vi "DP-Transpose.vi"(5 "USER ID":string="ML", 7 "ANIMAL ID":i32=15, 9 "EAR":string="R", 11 "RUN":i32, 13 "Array of f2's":i32[](array[numeric])=[5660, 6730, 8000, 9520, 11300, 13460, 16000, 19040, 22650, 26920, 32000, 38050, 45200]) -> ()   [LabVIEW 2020]
uses:
  <vilib>/Analysis/NI_AALBase.lvlib
panel:
  out "ERROR":bool
  in  "Criterion for Database":u16(ring)=1 items=["-5 dB", "0 dB ", "5 dB", "10 dB"]
  in  "Return":bool
  in  "Start":bool
  out "File Error":bool
  in  "PARTITION":string="C:\\Data\\"
  out "FINAL GRAPH":cluster{dbl[], dbl[]}[](graph)=[{[5.6, 22.6, 32.0], [72.77611940298507, 24.79591836734694, 35.338770388958594]}, {[5.6, 8.0, 16.0, 22.6, 32.0, 45.2], [85.0, 75.33814247069432, 32.34341252699784, 29.006462035541194, 38.47553324968632, 45.006435006435005]}, {[5.6, 8.0, 11.3, 16.0, 22.6, 32.0, 45.2], [85.0, 77.59242560865644, 77.35252808988764, 37.61316872427984, 33.12603648424544, 42.6440329218107, 48.22393822393823]}, {[5.6, 8.0, 11.3, 16.0, 22.6, 32.0, 45.2], [85.0, 79.84670874661857, 85.0, 43.13084112149533, 37.5607476635514, 50.080906148867314, 51.63265306122449]}, {[5.6, 8.0, 11.3, 16.0, 22.6, 32.0, 45.2], [85.0, 85.0, 85.0, 49.28211586901763, 43.80573248407644, 70.90986394557824, 55.329861111111114]}, {[5.6, 8.0, 11.3, 16.0, 22.6, 32.0, 45.2], [85.0, 85.0, 85.0, 57.552742616033754, 66.34316770186335, 72.32709750566893, 59.67013888888889]}, {[5.6, 8.0, 11.3, 16.0, 22.6, 32.0, 45.2], [85.0, 85.0, 85.0, 64.66019417475728, 70.18613607188703, 73.74433106575964, 65.31879194630872]}]
  in  "Which DP":bool=TRUE
  out "I-O GRAPH":cluster{ext[], ext[]}[](graph)=[{[10.0, 15.0, 20.0, 25.0, 30.0, 35.0, 40.0, 45.0, 50.0, 55.0, 60.0, 65.0, 70.0, 75.0, 80.0], [-21.38, -4.92, -4.57, -12.49, -18.58, -19.55, -10.63, -13.68, -10.35, -11.85, -9.81, -9.89, -6.86, -3.51, -9.21]}, {[10.0, 15.0, 20.0, 25.0, 30.0, 35.0, 40.0, 45.0, 50.0, 55.0, 60.0, 65.0, 70.0, 75.0, 80.0], [-12.46, -6.43, -7.62, 0.71, -8.47, -7.75, -3.16, -1.91, -3.14, -2.22, -12.37, -7.72, -2.6, -0.75, 10.34]}, {[10.0, 15.0, 20.0, 25.0, 30.0, 35.0, 40.0, 45.0, 50.0, 55.0, 60.0, 65.0, 70.0, 75.0, 80.0], [-9.79, -1.17, -1.26, 8.27, -8.03, -2.71, -6.35, -10.3, -1.88, -1.74, 0.93, 4.21, 2.16, 1.65, 8.77]}, {[10.0, 15.0, 20.0, 25.0, 30.0, 35.0, 40.0, 45.0, 50.0, 55.0, 60.0, 65.0, 70.0, 75.0, 80.0], [-6.83, -9.43, -10.07, -8.11, -2.17, 2.46, 7.32, 11.6, 15.57, 18.79, 21.16, 25.28, 30.33, 35.66, 37.1]}, {[10.0, 15.0, 20.0, 25.0, 30.0, 35.0, 40.0, 45.0, 50.0, 55.0, 60.0, 65.0, 70.0, 75.0, 80.0], [-9.81, -5.62, -5.94, -4.96, 1.23, 7.26, 12.61, 15.75, 17.7, 18.3, 18.08, 18.27, 24.71, 32.5, 37.52]}, {[10.0, 15.0, 20.0, 25.0, 30.0, 35.0, 40.0, 45.0, 50.0, 55.0, 60.0, 65.0, 70.0, 75.0, 80.0], [-7.23, -10.81, -18.72, -21.87, -8.97, -5.54, 2.43, 7.29, 9.95, 13.04, 14.52, 12.51, 11.79, 29.43, 37.82]}, {[10.0, 15.0, 20.0, 25.0, 30.0, 35.0, 40.0, 45.0, 50.0, 55.0, 60.0, 65.0, 70.0, 75.0, 80.0], [-1.57, -13.83, -4.88, -2.53, -4.33, -8.02, -2.22, -0.01, 7.76, 14.62, 20.38, 24.81, 27.79, 30.32, 31.98]}]
  in  "?":ext[](array[numeric]) format="%.2f"
  out "?":string="5645\t-10.9\t2.6\r7995\t-5.6\t2.3\r11322\t-4.1\t4.1\r15991\t-8.0\t3.2\r22644\t-8.5\t1.6\r32012\t-10.4\t2.7\r45257\t-5.0\t2.4\r"
  # "85 dB means DP never reaches criterion"
  # "Nse Flr"
  # "f2 (Hz)"
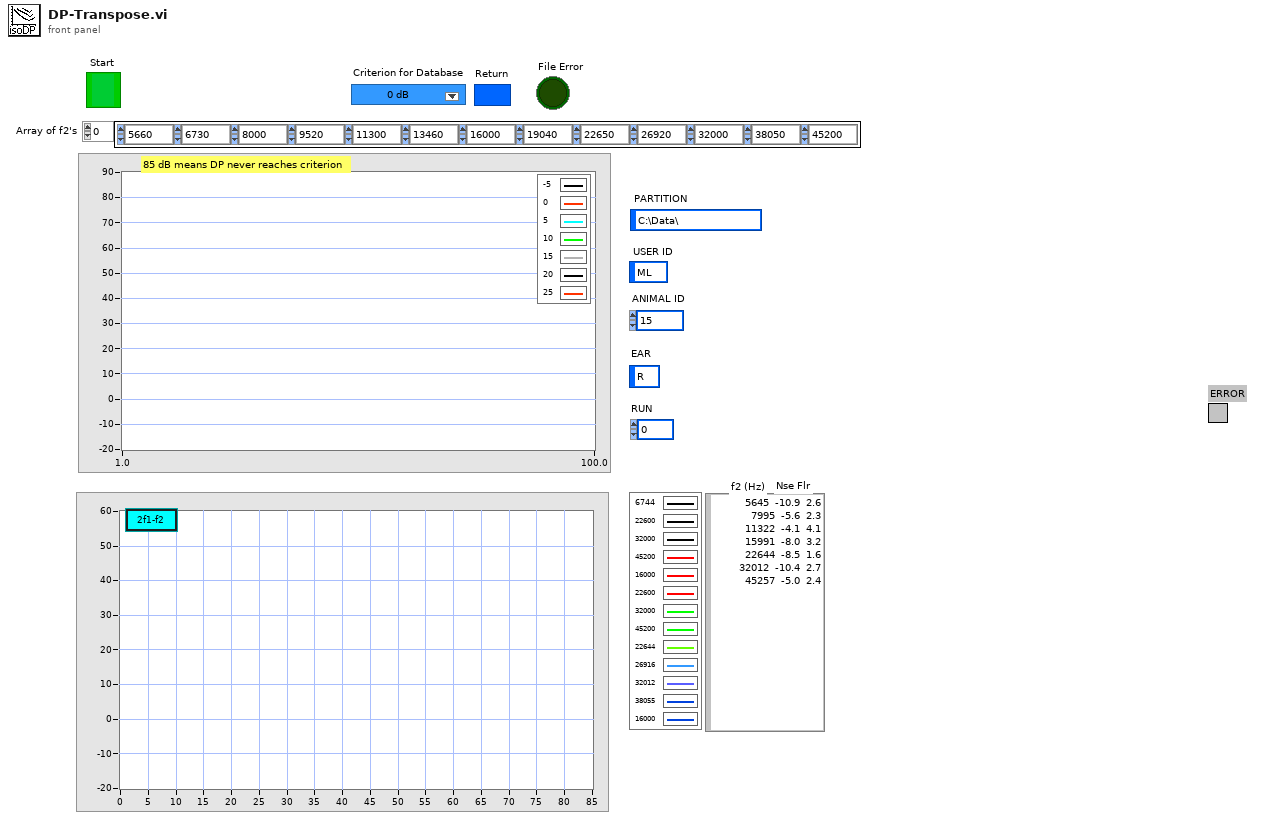
[diagram p1: front panel]
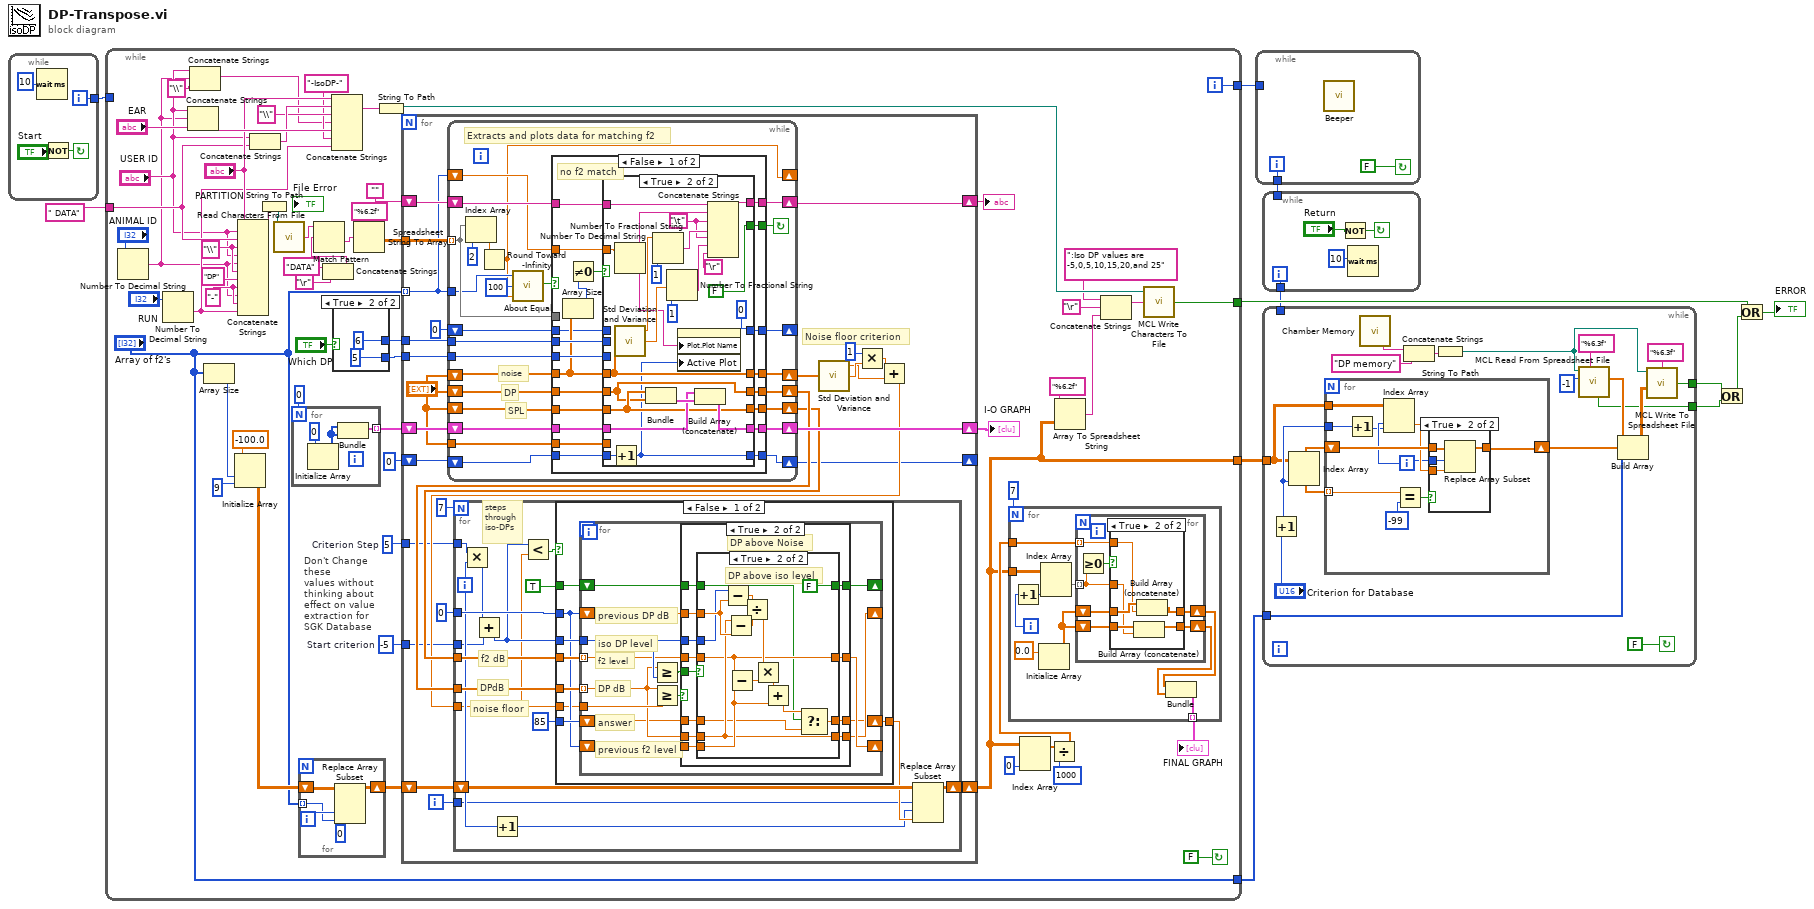
[diagram p0: block diagram]
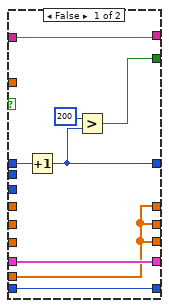
[diagram p4: hidden frame]
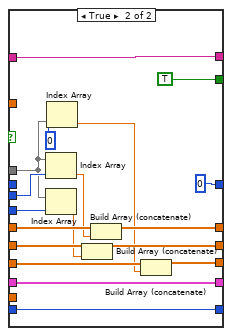
[diagram p5: hidden frame]
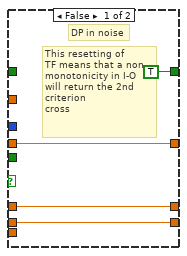
[diagram p6: hidden frame]
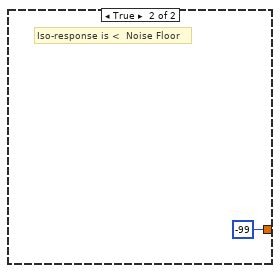
[diagram p8: hidden frame]
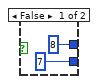
[diagram p9: hidden frame]
diagram:
  n1 = while {
    tunnel: [w16] -> w12
    i -> [w16]
    stop <- w14 continue-if-true
    n2 = Wait (ms)(milliseconds to wait=10) -> ()  [unwired: 1 out]
    n3 = Not(x="Start") -> (.not. x?=w14:bool)
  }
  n4 = while {
    tunnel: " DATA" -> [w29]
    tunnel: [w30] -> w4
    tunnel: w12 -> [_]
    tunnel: [w22] -> w10
    tunnel: [w17] -> w9
    tunnel: ["Array of f2's"] -> w1
    i -> [w30]
    stop <- FALSE continue-if-true
    w38 = 5  # Criterion Step
    w39 = -5  # Start criterion
    w71 = "-"
    w73 = "\\"
    # "Don't Change these\nvalues without thinking about\neffect on value extraction for\nSGK Database"
    n5 = Number To Decimal String(number="ANIMAL ID") -> (decimal integer string=w26:string)  [unwired: 1 in]
    n6 = Number To Decimal String(number="RUN") -> (decimal integer string=w28:string)  [unwired: 1 in]
    n7 = Concatenate Strings("USER ID", w26, "EAR") -> (w44:string)
    n8 = Concatenate Strings("USER ID", w26, "\\") -> (w24:string)
    n9 = Array Size(array="Array of f2's") -> (size(s)=w61:i32)
    n10 = Initialize Array(-100.0, w61, 9) -> (w57:dbl[][])
    n11 = Concatenate Strings("PARTITION", "USER ID", w29, w73, "USER ID", w26, w73, "DP", w71, w26, w71, w28) -> (w34:string)
    n12 = Concatenate Strings("USER ID", w29) -> (w42:string)
    n13 = String To Path(string=w34) -> (path=w70:path)
    n14 = call <vilib>:"Read Characters From File.vi"("file path (dialog if empty)"=w70) -> ("character string"=w33:string)  [unwired: 5 in, 3 out]
    n15 = for {
      N: 0 -> [_]
      tunnel: [w309] -> w63 mode=indexing
      n16 = Initialize Array(0) -> (w310:i32[])  [unwired: 1 in]
      n17 = Bundle(w310, w310) -> (w309:cluster{i32[], i32[]})  [unwired: 1 in]
    }
    n18 = for {
      shift-right: [w105] -> w58
      shift-left: w57 -> [w106]
      tunnel: "Array of f2's" -> [w102] mode=indexing
      i -> [w103]
      n19 = Replace Array Subset(array=w106, new element=w102, index (row)=w103, index (col)=0) -> (w105:dbl[][])
    }
    n20 = Concatenate Strings("DATA", "\r") -> (w35:string)
    n21 = Match Pattern(string=w33, regular expression=w35) -> (after substring=w32:string)  [unwired: 1 in, 3 out]
    n22 = Concatenate Strings("PARTITION", w42, "\\", w24, w44, "-IsoDP-", w28) -> (w23:string)
    n23 = case shown="True" "Which DP" {
      tunnel: [7 5] -> w76
      tunnel: [8 6] -> w75
      frame False {
      }
      frame True {
      }
    }
    n24 = Spreadsheet String To Array(format string="%6.2f", spreadsheet string=w32) -> (array=w21:dbl[][])  [unwired: 2 in]
    n25 = String To Path(string=w23) -> (path=w49:path)
    n26 = for {
      tunnel: w21 -> [w133]
      tunnel: w75 -> [w132]
      tunnel: w76 -> [w131]
      tunnel: "Array of f2's" -> [w110] mode=indexing
      shift-right: [w129] -> w59
      shift-left: "" -> [w130]
      shift-right: [w128] -> w64
      shift-left: w63 -> [w127]
      shift-right: [w123] -> w22
      shift-left: w58 -> [w124]
      tunnel: w39 -> [w113]
      tunnel: w38 -> [w112]
      shift-right: [w108] -> _
      shift-left: 0 -> [w109]
      i -> [w121]
      # "Noise floor criterion"
      n27 = while {
        shift-left: 0 -> [w137]
        shift-right: [w138] -> _
        shift-left: w110 -> [w142]
        shift-right: [w136] -> _
        tunnel: w110 -> [w140]
        shift-left: w127 -> [w145]
        shift-right: [w144] -> w128
        shift-left: w130 -> [w147]
        shift-right: [w148] -> w129
        tunnel: "?" -> [w149]
        tunnel: w131 -> [w150]
        tunnel: w132 -> [w151]
        shift-left: "?" -> [w153]
        shift-right: [w154] -> w120
        shift-left: "?" -> [w155]
        shift-right: [w156] -> w122
        shift-left: "?" -> [w157]
        shift-right: [w158] -> w119
        tunnel: w133 -> [w152] mode=indexing
        shift-right: [w135] -> w108
        shift-left: w109 -> [w134]
        stop <- w143 continue-if-true
        # "Extracts and plots data for matching f2"
        # "SPL"
        # "DP"
        # "noise"
        n28 = Index Array(array=w152, index=2) -> (element=w146:dbl)
        n29 = Round Toward -Infinity(1:w146) -> (0:w136:dbl)
        n30 = call "About Equal.vi"("Standard Value"=w136, "+/- Range"=100, "Input Value"=w140) -> ("In Range?"=w141:bool)
        n31 = case shown="False" w141 {
          tunnel: [w171 w222] -> w158
          tunnel: w157 -> [w165 w221]
          tunnel: [w172 w223] -> w156
          tunnel: w155 -> [w177 w220]
          tunnel: [w174 w224] -> w154
          tunnel: w153 -> [w178 w219]
          tunnel: w152 -> [_ w226]
          tunnel: w151 -> [w168 w228]
          tunnel: w150 -> [w169 w227]
          tunnel: w149 -> [w173 _]
          tunnel: [w180 w215] -> w148
          tunnel: w147 -> [w179 w215]
          tunnel: w145 -> [w176 w214]
          tunnel: [w175 w214] -> w144
          tunnel: [w170 TRUE] -> w143
          tunnel: w142 -> [w164 _]
          tunnel: [w163 0] -> w138
          tunnel: w137 -> [w162 _]
          tunnel: [w161 w211] -> w135
          tunnel: w134 -> [w160 w211]
          frame False {
            # "no f2 match"
            n32 = Array Size(array=w165) -> (size(s)=w167:i32)
            n33 = Not Equal To 0?(x=w167) -> (x != 0?=w166:bool)
            n34 = case shown="True" w166 {
              tunnel: [w187 w207] -> w175
              tunnel: w176 -> [w187 w206]
              tunnel: w177 -> [_ w201]
              tunnel: w178 -> [_ w202]
              tunnel: w179 -> [w188 w204]
              tunnel: [w188 w205] -> w180
              tunnel: w165 -> [_ w200]
              tunnel: [w186 w202] -> w174
              tunnel: w173 -> [w186 _]
              tunnel: [w186 w201] -> w172
              tunnel: [w186 w200] -> w171
              tunnel: [w183 FALSE] -> w170
              tunnel: w169 -> [_ _]
              tunnel: w168 -> [_ _]
              tunnel: w164 -> [_ w192]
              tunnel: [w184 0] -> w163
              tunnel: w162 -> [w185 _]
              tunnel: [w181 w190] -> w161
              tunnel: w160 -> [w181 w191]
              frame False {
                n35 = Increment(x=w185) -> (x+1=w184:i32)
                n36 = Greater?(x=200, y=w184) -> (0:w183:bool)
              }
              frame True {
                w196 = "\t"
                n37 = Increment(x=w191) -> (x+1=w190:i32)
                n38 = Number To Decimal String(number=w192) -> (decimal integer string=w189:string)  [unwired: 1 in]
                n39 = call <vilib>:"Std Deviation and Variance.vi"("X"=w200) -> ("mean"=w199:dbl, "standard deviation"=w197:dbl)  [unwired: 1 in, 1 out]
                n40 = Bundle(w202, w201) -> (w210:cluster{ext[], ext[]})  [unwired: 1 in]
                n41 = Number To Fractional String(number=w199, precision (6)=1) -> (F-format string=w209:string)  [unwired: 2 in]
                n42 = Number To Fractional String(number=w197, precision (6)=1) -> (F-format string=w195:string)  [unwired: 2 in]
                n43 = property on="I-O GRAPH" class="XYGraph (strict)"("Plot.Plot Name"=w189, "Active Plot"=w190) -> ()  [unwired: 2 in, 2 out]
                n44 = Build Array (concatenate)(w206, w210) -> (w207:cluster{ext[], ext[]}[])
                n45 = Concatenate Strings(w204, w189, w196, w209, w196, w195, "\r") -> (w205:string)
              }
            }
          }
          frame True {
            # "f2 match"
            n46 = Index Array(array=w226, index=w228) -> (element=w217:dbl)
            n47 = Index Array(array=w226, index=w227) -> (element=w216:dbl)
            n48 = Index Array(array=w226, index=0) -> (element=w218:dbl)
            n49 = Build Array (concatenate)(w220, w216) -> (w223:ext[])
            n50 = Build Array (concatenate)(w221, w217) -> (w222:ext[])
            n51 = Build Array (concatenate)(w219, w218) -> (w224:ext[])
          }
        }
      }
      n52 = call <vilib>:"Std Deviation and Variance.vi"("X"=w119) -> ("mean"=w115:dbl, "standard deviation"=w118:dbl)  [unwired: 1 in, 1 out]
      n53 = Multiply(x=1, y=w118) -> (x*y=w116:dbl)
      n54 = Add(x=w116, y=w115) -> (x+y=w114:dbl)
      n55 = for {
        N: 7 -> [_]
        tunnel: w114 -> [w229]
        tunnel: 0 -> [w245]
        tunnel: w122 -> [w244]
        shift-right: [w238] -> w123
        shift-left: w124 -> [w240]
        tunnel: w121 -> [w236]
        tunnel: w120 -> [w243]
        tunnel: w113 -> [w233]
        tunnel: w112 -> [w232]
        i -> [w239]
        # "noise floor"
        # "DPdB"
        # "f2 dB"
        # "steps through iso-DPs"
        n56 = Multiply(x=w232, y=w239) -> (x*y=w242:i32)
        n57 = Add(x=w242, y=w233) -> (x+y=w230:i32)
        n58 = Increment(x=w239) -> (x+1=w235:i32)
        n59 = Less?(x=w230, y=w229) -> (x < y?=w231:bool)
        n60 = case shown="False" w231 {
          tunnel: TRUE -> [w253 _]
          tunnel: [w252 -99] -> w237
          tunnel: 85 -> [w251 _]
          tunnel: w230 -> [w250 _]
          tunnel: w243 -> [w249 _]
          tunnel: w244 -> [w248 _]
          tunnel: w245 -> [w247 _]
          tunnel: w229 -> [w246 _]
          frame False {
            n61 = for {
              tunnel: w248 -> [w258] mode=indexing
              tunnel: w246 -> [w267]
              shift-right: [w264] -> _
              shift-left: w247 -> [w261]
              shift-right: [w263] -> _
              shift-left: w247 -> [w262]
              tunnel: w250 -> [w260]
              tunnel: w249 -> [w259] mode=indexing
              shift-right: [w256] -> w252
              shift-left: w251 -> [w257]
              shift-right: [w255] -> _
              shift-left: w253 -> [w254]
              # "DP dB"
              # "f2 level"
              # "answer"
              # "iso DP level"
              # "previous f2 level"
              # "previous DP dB"
              n62 = Greater Or Equal?(x=w258, y=w260) -> (x >= y?=w266:bool)
              n63 = Greater Or Equal?(x=w258, y=w267) -> (x >= y?=w265:bool)
              n64 = case shown="True" w265 {
                tunnel: w266 -> [_ w276]
                tunnel: w259 -> [w270 w283]
                tunnel: w258 -> [w271 w282]
                tunnel: [w270 w280] -> w264
                tunnel: [w271 w281] -> w263
                tunnel: w260 -> [_ w279]
                tunnel: w262 -> [_ w278]
                tunnel: w261 -> [_ w277]
                tunnel: w257 -> [w269 w274]
                tunnel: [w269 w275] -> w256
                tunnel: [TRUE w273] -> w255
                tunnel: w254 -> [_ w272]
                frame False {
                  # "This resetting of\nTF means that a non-\nmonotonicity in I-O\nwill return the 2nd\ncriterion\ncross"
                  # "DP in noise"
                }
                frame True {
                  # "DP above Noise"
                  n65 = case shown="True" w276 {
                    tunnel: w283 -> [w287 w293]
                    tunnel: w282 -> [w286 w294]
                    tunnel: [w286 w294] -> w281
                    tunnel: [w287 w293] -> w280
                    tunnel: w279 -> [_ w295]
                    tunnel: w278 -> [_ w296]
                    tunnel: w277 -> [_ w302]
                    tunnel: [w285 w291] -> w275
                    tunnel: w274 -> [w285 w289]
                    tunnel: [w284 FALSE] -> w273
                    tunnel: w272 -> [w284 w288]
                    frame False {
                      # "DP too small"
                    }
                    frame True {
                      # "DP above iso level"
                      n66 = Subtract(x=w295, y=w296) -> (x-y=w297:ext)
                      n67 = Subtract(x=w294, y=w296) -> (x-y=w298:ext)
                      n68 = Subtract(x=w293, y=w302) -> (x-y=w300:ext)
                      n69 = Divide(x=w297, y=w298) -> (x/y=w299:ext)
                      n70 = Multiply(x=w299, y=w300) -> (x*y=w301:ext)
                      n71 = Add(x=w301, y=w302) -> (x+y=w290:ext)
                      n72 = Select(t=w290, s=w288, f=w289) -> (s? t:f=w291:ext)
                    }
                  }
                }
              }
            }
          }
          frame True {
            # "Iso-response is <  Noise Floor"
          }
        }
        n73 = Replace Array Subset(array=w240, new element=w237, index (row)=w236, index (col)=w235) -> (w238:dbl[][])
      }
    }
    "I-O GRAPH" <- w64
    "?" <- w59
    n74 = Index Array(array=w22, index (col)=0) -> (element=w53:dbl[])  [unwired: 1 in]
    n75 = Divide(x=w53, y=1000) -> (x/y=w51:dbl[])
    n76 = for {
      N: 7 -> [_]
      tunnel: [w81] -> w55 mode=indexing
      tunnel: w22 -> [w80]
      tunnel: w51 -> [w77]
      i -> [w86]
      n77 = Increment(x=w86) -> (x+1=w83:i32)
      n78 = Initialize Array(0.0) -> (w78:dbl[])  [unwired: 1 in]
      n79 = Index Array(array=w80, index (col)=w83) -> (element=w85:dbl[])  [unwired: 1 in]
      n80 = for {
        shift-right: [w92] -> w82
        shift-left: w78 -> [w91]
        shift-right: [w90] -> w84
        shift-left: w78 -> [w89]
        tunnel: w85 -> [w87] mode=indexing
        tunnel: w77 -> [w88] mode=indexing
        n81 = Greater Or Equal To 0?(x=w87) -> (x >= 0?=w93:bool)
        n82 = case shown="True" w93 {
          tunnel: [w95 w100] -> w92
          tunnel: w91 -> [w95 w101]
          tunnel: [w94 w99] -> w90
          tunnel: w89 -> [w94 w98]
          tunnel: w88 -> [_ w97]
          tunnel: w87 -> [_ w96]
          frame False {
          }
          frame True {
            n83 = Build Array (concatenate)(w98, w96) -> (w99:dbl[])
            n84 = Build Array (concatenate)(w101, w97) -> (w100:dbl[])
          }
        }
      }
      n85 = Bundle(w82, w84) -> (w81:cluster{dbl[], dbl[]})  [unwired: 1 in]
    }
    "FINAL GRAPH" <- w55
    n86 = Array To Spreadsheet String(array=w22, 3:"%6.2f") -> (spreadsheet string=w47:string)  [unwired: 1 in]
    n87 = Concatenate Strings(":Iso DP values are -5,0,5,10,15,20,and 25", "\r", w47) -> (w48:string)
    n88 = call "MCL Write Characters To File.vi"("character string"=w48, "file path (dialog if empty)"=w49) -> ("Filewrite Error"=w17:bool)  [unwired: 2 in, 1 out]
  }
  n89 = while {
    tunnel: w4 -> [_]
    tunnel: [w312] -> w3
    i -> [w312]
    stop <- FALSE continue-if-true
    n90 = call "Beeper.vi"() -> ()  [unwired: 1 in]
  }
  n91 = while {
    tunnel: w3 -> [_]
    tunnel: [w313] -> w2
    i -> [w313]
    stop <- w315 continue-if-true
    n92 = Not(x="Return") -> (.not. x?=w315:bool)
    n93 = Wait (ms)(milliseconds to wait=10) -> ()  [unwired: 1 out]
  }
  n94 = while {
    tunnel: w10 -> [w318]
    tunnel: [w324] -> w6
    tunnel: [w317] -> w5
    tunnel: w2 -> [_]
    tunnel: w1 -> [w322]
    stop <- FALSE continue-if-true
    n95 = Increment(x="Criterion for Database") -> (x+1=w320:u16)
    n96 = Index Array(array=w318, index (col)=w320) -> (element=w319:dbl[])  [unwired: 1 in]
    n97 = for {
      shift-right: [w341] -> w321
      shift-left: w319 -> [w340]
      tunnel: w319 -> [w343] mode=indexing
      tunnel: w318 -> [w339]
      tunnel: w320 -> [w338]
      i -> [w336]
      n98 = Increment(x=w338) -> (x+1=w335:u16)
      n99 = Index Array(array=w339, index (row)=w336, index (col)=w335) -> (element=w337:dbl)
      n100 = Equal?(x=w343, y=-99) -> (x = y?=w342:bool)
      n101 = case shown="True" w342 {
        tunnel: [w345 w348] -> w341
        tunnel: w340 -> [w345 w349]
        tunnel: w336 -> [_ w347]
        tunnel: w337 -> [_ w346]
        frame False {
        }
        frame True {
          n102 = Replace Array Subset(array=w349, new element=w346, index=w347) -> (w348:dbl[])
        }
      }
    }
    n103 = call "Chamber Memory.vi"() -> ("Filepath for Memory Bank"=w333:string)  [unwired: 3 in, 3 out]
    n104 = Concatenate Strings(w333, "DP memory") -> (w332:string)
    n105 = String To Path(string=w332) -> (path=w325:path)
    n106 = call "MCL Read From Spreadsheet File.vi"("format (%.3f)"="%6.3f", "number of rows (all:-1)"=-1, "file path (dialog if empty)"=w325) -> ("first row"=w328:sgl[], "Fileread Error"=w317:bool)  [unwired: 3 in, 4 out]
    n107 = Build Array(w328, w321, w322) -> (w326:dbl[][])
    n108 = call "MCL Write To Spreadsheet File.vi"("format (%.3f)"="%6.3f", "2D data"=w326, "file path (dialog if empty)"=w325) -> ("Filesave Error"=w324:bool)  [unwired: 4 in, 1 out]
  }
  n109 = Or(x=w6, y=w5) -> (x .or. y?=w7:bool)
  n110 = Or(x=w9, y=w7) -> (x .or. y?=→"ERROR":bool)
